vi "Adjust Spacing and Visibility.vi"(0 "Cluster Ref Array":refnum<vi>[](array[refnum]), 2 "Position Index":i32, 11 "Sub Panel Ref Array":refnum<vi>[](array[refnum])) -> (15 "Sub Panel Ref Array Dup":refnum<vi>[](array[refnum]))   [LabVIEW 2016]
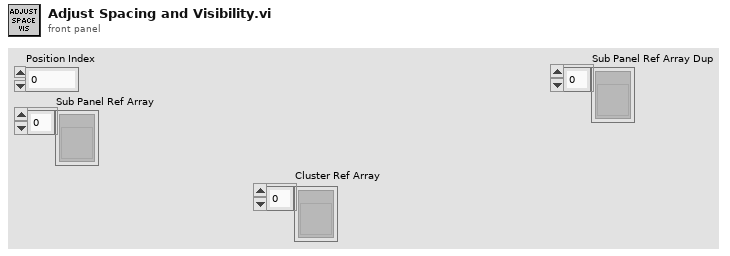
[diagram p1: front panel]
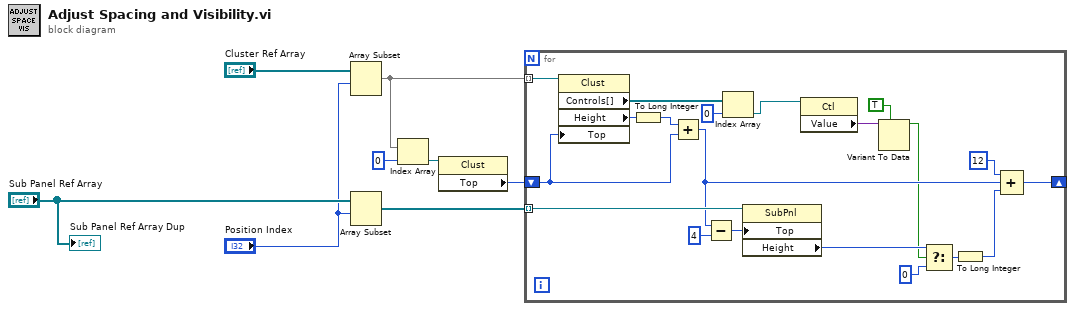
[diagram p0: block diagram]
diagram:
  n1 = Array Subset(array="Cluster Ref Array", index="Position Index") -> (w4:refnum<vi>[])  [unwired: 1 in]
  n2 = Array Subset(array="Sub Panel Ref Array", index="Position Index") -> (w5:refnum<vi>[])  [unwired: 1 in]
  n3 = Index Array(array=w4, index=0) -> (element=w2:refnum<vi>)
  n4 = property class="Clust"(reference=w2) -> ("Top"=w1:i32)  [unwired: 1 in, 2 out]
  n5 = for {
    tunnel: w4 -> [w28] mode=indexing
    tunnel: w5 -> [w25] mode=indexing
    shift-right: [w19] -> _
    shift-left: w1 -> [w16]
    n6 = property class="Clust"(reference=w28, "Top"=w16) -> ("Controls[]"=w14:refnum<vi>[], "Height"=w27:u32)  [unwired: 1 in, 2 out]
    n7 = To Long Integer(number=w27) -> (32bit integer=w26:i32)
    n8 = Add(x=w26, y=w16) -> (x+y=w15:i32)
    n9 = Subtract(x=w15, y=4) -> (x-y=w23:i32)
    n10 = Index Array(array=w14, index=0) -> (element=w12:refnum<vi>)
    n11 = property class="SubPnl"(reference=w25, "Top"=w23) -> ("Height"=w22:u32)  [unwired: 1 in, 2 out]
    n12 = property class="Ctl"(reference=w12) -> ("Value"=w11:variant)  [unwired: 1 in, 2 out]
    n13 = Variant To Data(type=TRUE, Variant=w11) -> (data=w9:bool)  [unwired: 1 in, 1 out]
    n14 = Select(t=w22, s=w9, f=u32 0) -> (s? t:f=w20:u32)
    n15 = To Long Integer(number=w20) -> (32bit integer=w17:i32)
    n16 = Compound Arithmetic op=ADD(12 ("x"), w15, w17) -> (w19:i32)
  }
  "Sub Panel Ref Array Dup" <- "Sub Panel Ref Array"
